vi "Process.vi"(8 "error in (no error)":errorcluster, 10 "Pound in":refnum<class "Pound.lvclass">, 11 "Qbus in":refnum<class "Qbus.lvclass">) -> (0 "error out":errorcluster)   [LabVIEW 2017, in "IrTestPanel.lvlib"]
uses:
  <vilib>/addons/InsightCM/Devices/Shared/Ir/IrTestPanel/IrTestPanel.lvlib
  <vilib>/addons/Qbus/Qbus.lvclass
  <vilib>/NI/Software Watchdog/Pound/Pound.lvclass
  <vilib>/addons/InsightCM/Devices/Shared/Ir/IrTestPanel/controls/config.ctl
  <vilib>/addons/InsightCM/Devices/Shared/Common/TestPanel/controls/Configuration.ctl
  <vilib>/addons/InsightCM/Devices/Shared/Common/TestPanel/controls/State.ctl
  <vilib>/addons/InsightCM/MessageBus/Base/controls/IRoutingSource.ctl
  <vilib>/NI/Software Watchdog/Watchdog/Watchdog.lvclass
  <vilib>/addons/InsightCM/Devices/Shared/Common/DataFlow/DataFlow.lvlib
  <vilib>/addons/InsightCM/Utilities/GlobalConfiguration/GlobalConfiguration.lvlib
  <vilib>/addons/TraceLogger/TraceLogger.lvlib
  <vilib>/addons/InsightCM/Devices/Shared/Common/TestPanel/TestPanel.lvlib
  <vilib>/addons/InsightCM/Devices/Shared/Common/ServerComm/ServerComm.lvlib
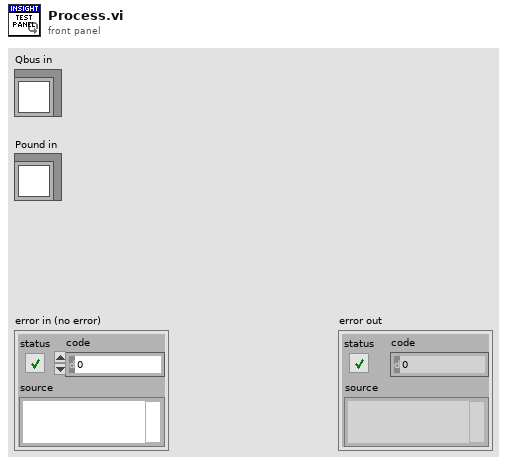
[diagram p1: front panel]
types:
  T1 = typedef "IrTestPanel.lvlib/config.ctl" = cluster{"Common":T2, "CameraInfo":variant}
  T2 = typedef "TestPanel.lvlib/Configuration.ctl" = cluster{"State":T3, "Waveform Channel":string, "DataGroup":string, "Number of Samples":i32, "Timeout":dbl, "History":variant, "LastRequest":timestamp, "BufferSize":i32, "OpState":variant, "IRoutingSource":T4}
  T3 = typedef "TestPanel.lvlib/State.ctl" = enum16{"Off", "On", "PendingValues", "PendingDataSet"}
  T4 = typedef "IRoutingSource.ctl" = cluster{"CorrelationId":string, "ReplyTo":string}
  T5 = typedef "DataFlow.lvlib/Data.ctl" = cluster{"DataGroup":string, "Waveforms":T6, "Map":T7, "Type":T8}
  T6 = typedef "wfmSGL_DVR.ctl" = refnum<data-value>
  T7 = typedef "PointValueMap.lvlib/PointMap.ctl" = refnum<data-value>
  T8 = typedef "DataFlow.lvlib/Type.ctl" = enum16{"High Rate", "Low Rate", "Burst Mode"}
  T9 = typedef "Message.ctl" = cluster{"Header":T10, "Body":u8[]}
  T10 = typedef "MessageHeader.ctl" = cluster{"MessageName":string, "Timestamp":i64, "CorrelationId":string, "ContentType":string, "RoutingKey":string, "Properties":T11[]}
  T11 = typedef "KeyValuePair.ctl" = cluster{"Key":string, "Value":string}
  T12 = typedef "DeviceTestPanelGetTimeSeriesRequestBody.ctl" = cluster{"DataGroup":string, "TrendPointIds":string[]}
  T13 = typedef "DeviceTestPanelGetDataSetForChannelRequestBody.ctl" = cluster{"DataGroup":string, "ChannelName":string, "Properties":T11[]}
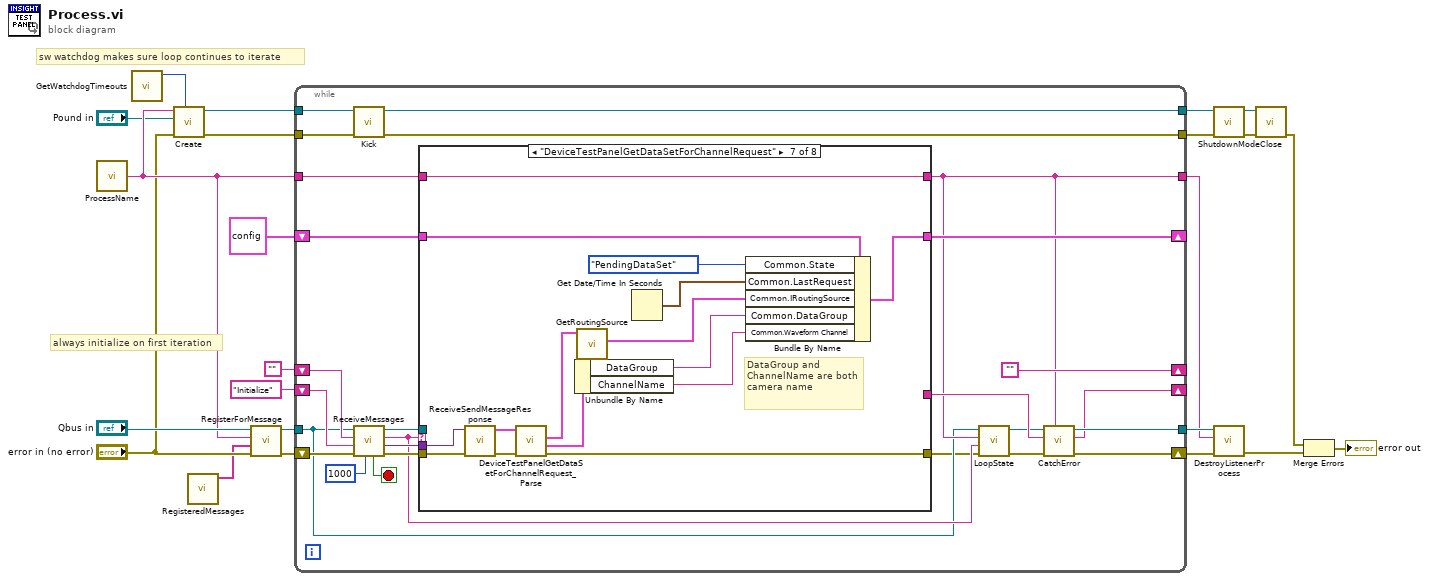
[diagram p0: block diagram]
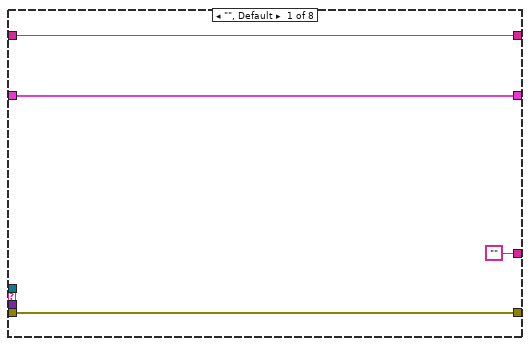
[diagram p2: hidden frame]
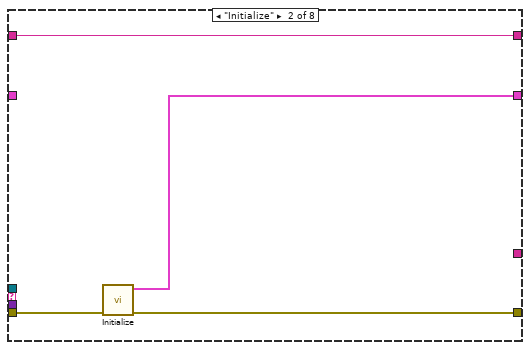
[diagram p3: hidden frame]
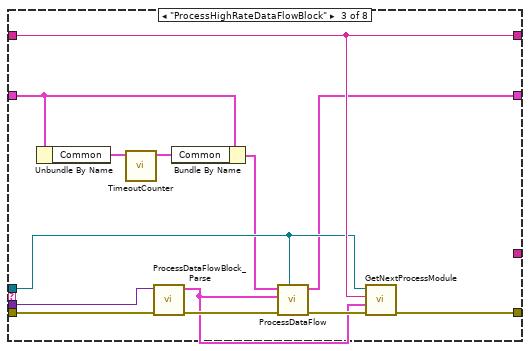
[diagram p4: hidden frame]
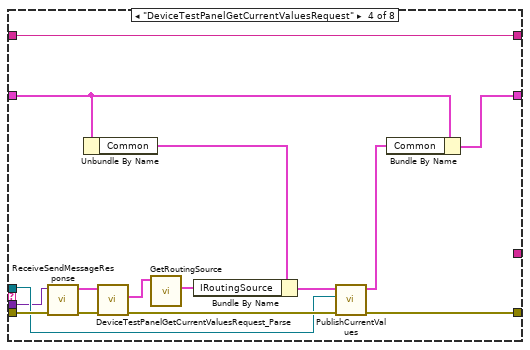
[diagram p5: hidden frame]
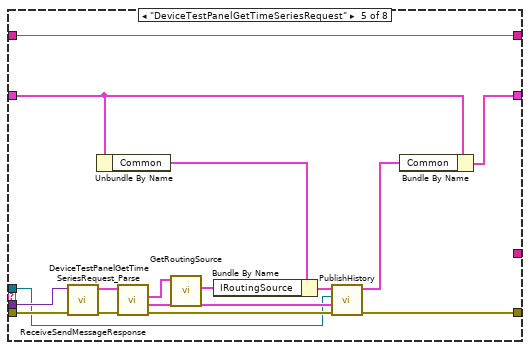
[diagram p6: hidden frame]
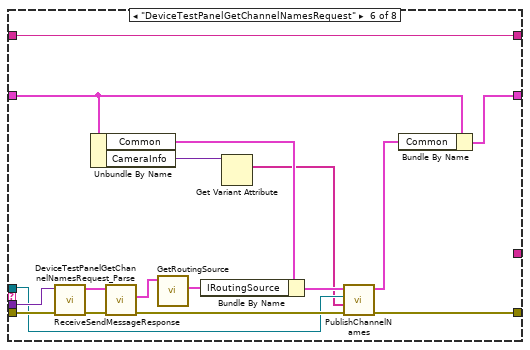
[diagram p7: hidden frame]
diagram:
  # "always initialize on first iteration"
  # "sw watchdog makes sure loop continues to iterate"
  n1 = call <vilib>:"ProcessName.vi"() -> ("process name"=w15:string)  [unwired: 5 in]
  n2 = call <vilib>:"GetWatchdogTimeouts.vi"() -> ("software timeout"=w3:u32)  [unwired: 10 in, 1 out]
  n3 = call <vilib>:"Create.vi"("Execution Timeout (ms)"=w3, "error in (no error)"="error in (no error)", "Pound"="Pound in", "Name"=w15) -> ("error out"=w9:errorcluster, "Watchdog"=w14:refnum<data-value>)  [unwired: 6 in]
  n4 = call <vilib>:"RegisteredMessages.vi"() -> ("registered messages"=w1:string[])  [unwired: 11 in]
  n5 = call <vilib>:"RegisterForMessage.vi"("error in (no error)"="error in (no error)", "message names"=w1, "process name"=w15, "Qbus in"="Qbus in") -> ("error in (no error)"=w22:errorcluster, "Qbus out"=w21:refnum<class "Qbus.lvclass">)  [unwired: 6 in]
  n6 = while {
    shift-right: [""] -> _
    shift-left: "" -> [w48]
    tunnel: w21 -> [w27]
    tunnel: w15 -> [w31]
    tunnel: [w39] -> w19
    tunnel: [w28] -> w18
    shift-right: [w38] -> _
    shift-left: "Initialize" -> [w43]
    shift-right: [w41] -> _
    shift-left: T1 {"Common"={"State"=enum."Off", "Waveform Channel"="", "DataGroup"="", "Number of Samples"=0, "Timeout"=0.0, "History"=variant, "LastRequest"=timestamp(0 s since 1904-01-01), "BufferSize"=0, "OpState"=variant, "IRoutingSource"={"CorrelationId"="", "ReplyTo"=""}}, "CameraInfo"=variant(string[] [])} ("config") -> [w42]
    tunnel: w14 -> [w37]
    tunnel: [w36] -> w11
    tunnel: w9 -> [w35]
    tunnel: [w33] -> w8
    shift-right: [w40] -> w20
    shift-left: w22 -> [w34]
    stop <- w49 stop-if-true
    n7 = call <vilib>:"Kick.vi"("error in (no error)"=w35, "Watchdog"=w37) -> ("error out"=w33:errorcluster, "Watchdog"=w36:refnum<data-value>)  [unwired: 8 in]
    n8 = call <vilib>:"ReceiveMessages.vi"("Timeout(1000)"=1000 ("milliseconds to wait"), "error in (no error)"=w34, "priority action"=w43, "default action"=w48, "Qbus in"=w27) -> ("error out"=w47:errorcluster, "message value"=w44:variant, "action"=w29:string, "Qbus out"=w45:refnum<class "Qbus.lvclass">, "exit"=w49:bool)  [unwired: 2 in]
    n9 = case shown="\"DeviceTestPanelGetDataSetForChannelRequest\"" w29 {
      tunnel: w47 -> [w50 w56 w69 w82 w96 w113 w125 w136]
      tunnel: w45 -> [_ _ w64 w77 w86 w104 _ _]
      tunnel: [w50 w55 w68 w75 w87 w109 w124 w136] -> w26
      tunnel: w44 -> [_ _ w70 w76 w95 w112 w122 _]
      tunnel: w42 -> [w53 _ w61 w73 w89 w106 w121 w135]
      tunnel: [w53 w54 w58 w72 w88 w105 w120 w135] -> w41
      tunnel: [w52 w57 w67 w71 w101 w118 w133 w134] -> w28
      tunnel: w31 -> [w52 w57 w67 w71 w101 w118 w133 w134]
      tunnel: ["" _ _ _ _ _ _ _] -> w30
      frame "", Default {
      }
      frame "Initialize" {
        n10 = call <vilib>:"Initialize.vi"("error in (no error)"=w56) -> ("error out"=w55:errorcluster, "config"=w54:T1)  [unwired: 9 in]
      }
      frame "ProcessHighRateDataFlowBlock" {
        n11 = Unbundle By Name(w61) -> ("Common"=w62:T2)
        n12 = call <vilib>:"TimeoutCounter.vi"("config in"=w62) -> ("config out"=w60:T2)  [unwired: 10 in]
        n13 = call <vilib>:"ProcessDataFlowBlock_Parse.vi"("error in (no error)"=w69, "body"=w70) -> ("error out"=w66:errorcluster, "data"=w63:T5)  [unwired: 8 in]
        n14 = Bundle By Name(cluster=w61, "Common"=w60) -> (w59:T1)
        n15 = call <vilib>:"ProcessDataFlow.vi"("Qbus in"=w64, "error in (no error)"=w66, "Data"=w63, "config in"=w59) -> ("error out"=w65:errorcluster, "config out"=w58:T1)  [unwired: 6 in]
        n16 = call <vilib>:"GetNextProcessModule.vi"("error in (no error)"=w65, "data"=w63, "source"=w67, "Qbus in"=w64) -> ("error out"=w68:errorcluster)  [unwired: 6 in, 1 out]
      }
      frame "DeviceTestPanelGetCurrentValuesRequest" {
        n17 = call <vilib>:"ReceiveSendMessageResponse.vi"("error in (no error)"=w82, "body"=w76) -> ("error out"=w81:errorcluster, "message"=w83:T9)  [unwired: 6 in, 2 out]
        n18 = Unbundle By Name(w73) -> ("Common"=w79:T2)
        n19 = call <vilib>:"DeviceTestPanelGetCurrentValuesRequest_Parse.vi"("error in (no error)"=w81, "Message"=w83) -> ("error out"=w80:errorcluster, "Header"=w84:T10)  [unwired: 7 in, 1 out]
        n20 = call <vilib>:"GetRoutingSource.vi"("Header in"=w84) -> ("IRoutingSource"=w85:T4)  [unwired: 9 in, 1 out]
        n21 = Bundle By Name(cluster=w79, "IRoutingSource"=w85) -> (w78:T2)
        n22 = call <vilib>:"PublishCurrentValues.vi"("error in (no error)"=w80, "Qbus in"=w77, "config in"=w78) -> ("error out"=w75:errorcluster, "config out"=w74:T2)  [unwired: 7 in]
        n23 = Bundle By Name(cluster=w73, "Common"=w74) -> (w72:T1)
      }
      frame "DeviceTestPanelGetTimeSeriesRequest" {
        n24 = call <vilib>:"ReceiveSendMessageResponse.vi"("error in (no error)"=w96, "body"=w95) -> ("error out"=w99:errorcluster, "message"=w98:T9)  [unwired: 6 in, 2 out]
        n25 = Unbundle By Name(w89) -> ("Common"=w94:T2)
        n26 = call <vilib>:"DeviceTestPanelGetTimeSeriesRequest_Parse.vi"("error in (no error)"=w99, "Message"=w98) -> ("error out"=w92:errorcluster, "Body"=w91:T12, "Header"=w97:T10)  [unwired: 6 in, 1 out]
        n27 = call <vilib>:"GetRoutingSource.vi"("Header in"=w97) -> ("IRoutingSource"=w100:T4)  [unwired: 9 in, 1 out]
        n28 = Bundle By Name(cluster=w94, "IRoutingSource"=w100) -> (w93:T2)
        n29 = call <vilib>:"PublishHistory.vi"("error in (no error)"=w92, "Body"=w91, "Qbus in"=w86, "config in"=w93) -> ("error out"=w87:errorcluster, "config out"=w90:T2)  [unwired: 6 in]
        n30 = Bundle By Name(cluster=w89, "Common"=w90) -> (w88:T1)
      }
      frame "DeviceTestPanelGetChannelNamesRequest" {
        n31 = call <vilib>:"ReceiveSendMessageResponse.vi"("error in (no error)"=w113, "body"=w112) -> ("error out"=w115:errorcluster, "message"=w116:T9)  [unwired: 6 in, 2 out]
        n32 = Unbundle By Name(w106) -> ("Common"=w111:T2, "CameraInfo"=w103:variant)
        n33 = call <vilib>:"DeviceTestPanelGetChannelNamesRequest_Parse.vi"("error in (no error)"=w115, "Message"=w116) -> ("error out"=w110:errorcluster, "Header"=w114:T10)  [unwired: 7 in, 1 out]
        n34 = call <vilib>:"GetRoutingSource.vi"("Header in"=w114) -> ("IRoutingSource"=w117:T4)  [unwired: 9 in, 1 out]
        n35 = Bundle By Name(cluster=w111, "IRoutingSource"=w117) -> (w108:T2)
        n36 = Get Variant Attribute(Variant=w103) -> (names=w102:string[])  [unwired: 3 in, 3 out]
        n37 = call <vilib>:"PublishChannelNames.vi"("error in (no error)"=w110, "names"=w102, "Qbus in"=w104, "config in"=w108) -> ("error out"=w109:errorcluster, "config out"=w107:T2)  [unwired: 6 in]
        n38 = Bundle By Name(cluster=w106, "Common"=w107) -> (w105:T1)
      }
      frame "DeviceTestPanelGetDataSetForChannelRequest" {
        # "DataGroup and ChannelName are both camera name"
        n39 = call <vilib>:"ReceiveSendMessageResponse.vi"("error in (no error)"=w125, "body"=w122) -> ("error out"=w131:errorcluster, "message"=w132:T9)  [unwired: 6 in, 2 out]
        n40 = call <vilib>:"DeviceTestPanelGetDataSetForChannelRequest_Parse.vi"("error in (no error)"=w131, "Message"=w132) -> ("error out"=w124:errorcluster, "Body"=w130:T13, "Header"=w128:T10)  [unwired: 6 in, 1 out]
        n41 = Unbundle By Name(w130) -> ("DataGroup"=w126:string, "ChannelName"=w123:string)
        n42 = call <vilib>:"GetRoutingSource.vi"("Header in"=w128) -> ("IRoutingSource"=w127:T4)  [unwired: 9 in, 1 out]
        n43 = Get Date/Time In Seconds() -> (seconds since 1Jan1904=w129:timestamp)
        n44 = Bundle By Name(cluster=w121, "Common.State"=State."PendingDataSet" ("Test Panel State"), "Common.LastRequest"=w129, "Common.IRoutingSource"=w127, "Common.DataGroup"=w126, "Common.Waveform Channel"=w123) -> (w120:T1)
      }
      frame "Exit" {
      }
    }
    n45 = call <vilib>:"LoopState.vi"("error in (no error)"=w26, "loop action"=w29, "process name"=w28, "Qbus in"=w27) -> ("error out"=w25:errorcluster, "Qbus out"=w24:refnum<class "Qbus.lvclass">)  [unwired: 6 in]
    n46 = call <vilib>:"CatchError.vi"("source"=w28, "error in (no error)"=w25, "next action in"=w30, "Qbus in"=w24) -> ("error out"=w40:errorcluster, "next action out"=w38:string, "Qbus out"=w39:refnum<class "Qbus.lvclass">)  [unwired: 5 in]
  }
  n47 = call <vilib>:"ShutdownMode.vi"("error in (no error)"=w8, "Watchdog"=w11) -> ("error out"=w10:errorcluster, "Watchdog"=w12:refnum<data-value>)  [unwired: 8 in]
  n48 = call <vilib>:"DestroyListenerProcess.vi"("error in (no error)"=w20, "process name"=w18, "Qbus in"=w19) -> ("error in (no error)"=w7:errorcluster)  [unwired: 7 in, 1 out]
  n49 = call <vilib>:"Close.vi"("error in (no error)"=w10, "Watchdog"=w12) -> ("error out"=w6:errorcluster)  [unwired: 9 in]
  n50 = Merge Errors(w6, w7) -> (→"error out":errorcluster)
